vi "PDF_FindData.vi"(10 "Code":string, 11 "Database Path":path) -> ()   [LabVIEW 2014]
uses:
  <vilib>/Utility/file.llb/Read From Spreadsheet File (string).vi
panel:
  out "all rows":string[][](array[string])
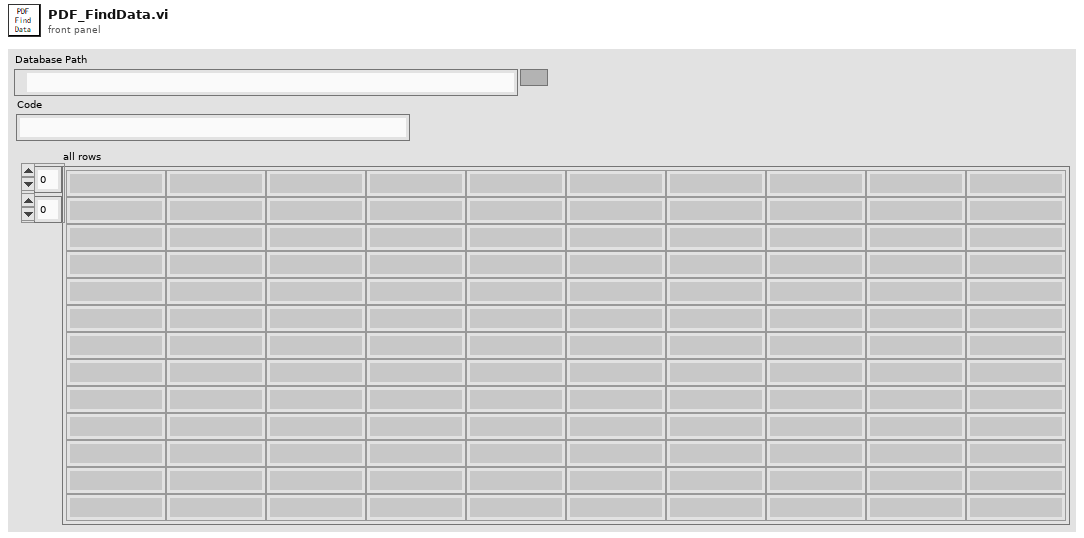
[diagram p1: front panel]
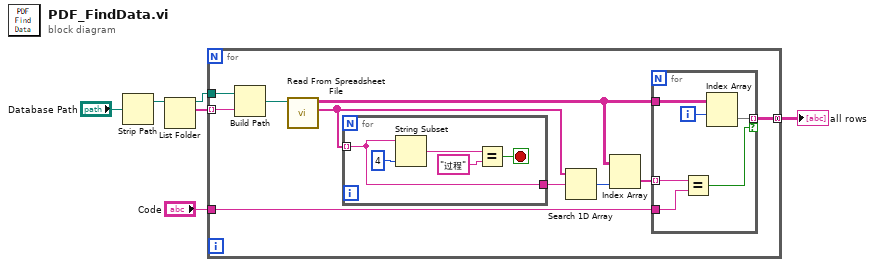
[diagram p0: block diagram]
diagram:
  n1 = Strip Path(path="Database Path") -> (stripped path=w3:path)  [unwired: 1 out]
  n2 = List Folder(path=w3) -> (path out=w5:path, filenames=w4:string[])  [unwired: 3 in, 2 out]
  n3 = for {
    tunnel: w5 -> [w16]
    tunnel: w4 -> [w15] mode=indexing
    tunnel: "Code" -> [w9]
    tunnel: [w7] -> w1 mode=concatenating
    n4 = Build Path(base path=w16, name or relative path=w15) -> (appended path=w13:path)
    n5 = call-poly <vilib>:"Read From Spreadsheet File.vi"("file path (dialog if empty)"=w13) -> ("first row"=w12:string[], "all rows"=w8:string[][])  [unwired: 6 in, 3 out]
    n6 = for {
      tunnel: w12 -> [w24] mode=indexing
      tunnel: [w24] -> w11
      stop <- w25 stop-if-true
      n7 = String Subset(string=w24, length (rest)=4 ("长度（剩余）")) -> (substring=w27:string)  [unwired: 1 in]
      n8 = Equal?(x=w27, y="过程" ("正则表达式")) -> (x = y?=w25:bool)
    }
    n9 = Search 1D Array(1D array=w12, element=w11) -> (index of element=w14:i32)  [unwired: 1 in]
    n10 = Index Array(array=w8, index (col)=w14) -> (element=w10:string[])  [unwired: 1 in]
    n11 = for {
      tunnel: w10 -> [w22] mode=indexing
      tunnel: w9 -> [w21]
      tunnel: w8 -> [w20]
      tunnel: [w18] -> w7 mode=indexing if=w17
      i -> [w19]
      n12 = Equal?(x=w22, y=w21) -> (x = y?=w17:bool)
      n13 = Index Array(array=w20, index (row)=w19) -> (element=w18:string[])  [unwired: 1 in]
    }
  }
  "all rows" <- w1
